vi "Tool Class Sandbox.vi"() -> ()   [LabVIEW 2011]
uses:
  Tool Class.lvclass
panel:
  out "error out":errorcluster
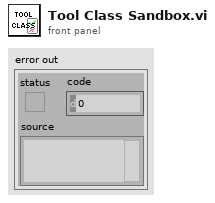
[diagram p1: front panel]
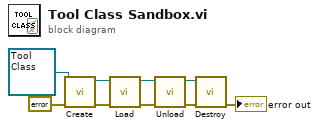
[diagram p0: block diagram]
diagram:
  n1 = call-dynamic "Create.vi"("error in (no error)"=errorcluster {"status"=FALSE, "code"=0, "source"=""} ("error constant"), "Tool Class in"=refnum<class "Tool Class.lvclass"> refnum) -> ("error out"=w7:errorcluster, "Tool Class out"=w6:refnum<class "Tool Class.lvclass">)  [unwired: 8 in]
  n2 = call-dynamic "Load.vi"("error in (no error)"=w7, "Tool Class in"=w6) -> ("error out"=w9:errorcluster, "Tool Class out"=w8:refnum<class "Tool Class.lvclass">)  [unwired: 8 in]
  n3 = call-dynamic "Unload.vi"("error in (no error)"=w9, "Tool Class in"=w8) -> ("error out"=w5:errorcluster, "Tool Class out"=w4:refnum<class "Tool Class.lvclass">)  [unwired: 8 in]
  n4 = call-dynamic "Destroy.vi"("error in (no error)"=w5, "Tool Class in"=w4) -> ("error out"=→"error out":errorcluster)  [unwired: 8 in, 1 out]
